vi "Config Relays.vi"(0 "VISA resource name":refnum<visa-resource-name>, 5 "Relay (1)":dbl=1.0 min=1.0 max=8.0 step=1.0, 7 "Input (1)":dbl=1.0 min=1.0 max=8.0 step=1.0, 9 "Mode (0:Off)":u16(ring) items=["Off", "On", "Alarms"], 11 "error in (no error)":errorcluster, 12 "Alarm Type (0:Off)":u16(ring) items=["Low", "High", "Both"]) -> (4 "VISA resource name out":refnum<visa-resource-name>, 15 "error out":errorcluster)   [LabVIEW 2017, in "Lake Shore Cryotronics 218.lvlib"]
doc: "This VI configures relay paramters. Relays may be configured manually or set to activate on an input alarm condition. Only the model 218S includes the relays."
uses:
  Lake Shore Cryotronics 218.lvlib
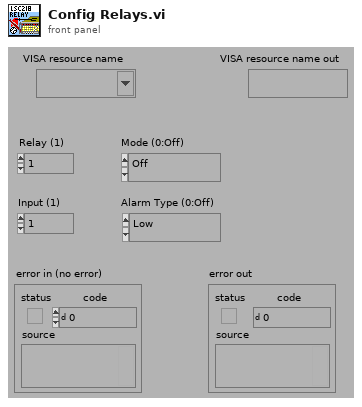
[diagram p1: front panel]
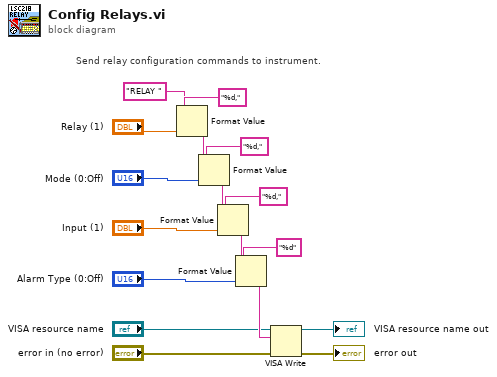
[diagram p0: block diagram]
diagram:
  # "Send relay configuration commands to instrument."
  n1 = Format Value(string ("")="RELAY ", format string="%d,", value (0)="Relay (1)") -> (output string=w12:string)
  n2 = Format Value(string ("")=w12, format string="%d,", value (0)="Mode (0:Off)") -> (output string=w11:string)
  n3 = Format Value(string ("")=w11, format string="%d,", value (0)="Input (1)") -> (output string=w7:string)
  n4 = Format Value(string ("")=w7, format string="%d", value (0)="Alarm Type (0:Off)") -> (output string=w5:string)
  n5 = VISA Write(VISA resource name="VISA resource name", write buffer=w5, error in (no error)="error in (no error)") -> (VISA resource name out=→"VISA resource name out":refnum<visa-resource-name>, error out=→"error out":errorcluster)  [unwired: 1 out]
